vi "占空比.vi"() -> (1 "T1+T2":dbl, 2 "T2":dbl, 3 "T1":dbl)   [LabVIEW 2020]
uses:
  <vilib>/DAQmx/read.llb/DAQmx Read (Counter 1D DBL 1Chan NSamp).vi
  <vilib>/DAQmx/create/channels.llb/DAQmx Create Channel (CI-Pulse Width).vi
  <vilib>/DAQmx/miscellaneous.llb/DAQmx Fill In Error Info.vi
  <vilib>/ptbypt/NI_PtbyPt.lvlib
  <resource>/objmgr/daqmx.rc
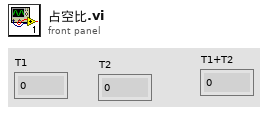
[diagram p1: front panel]
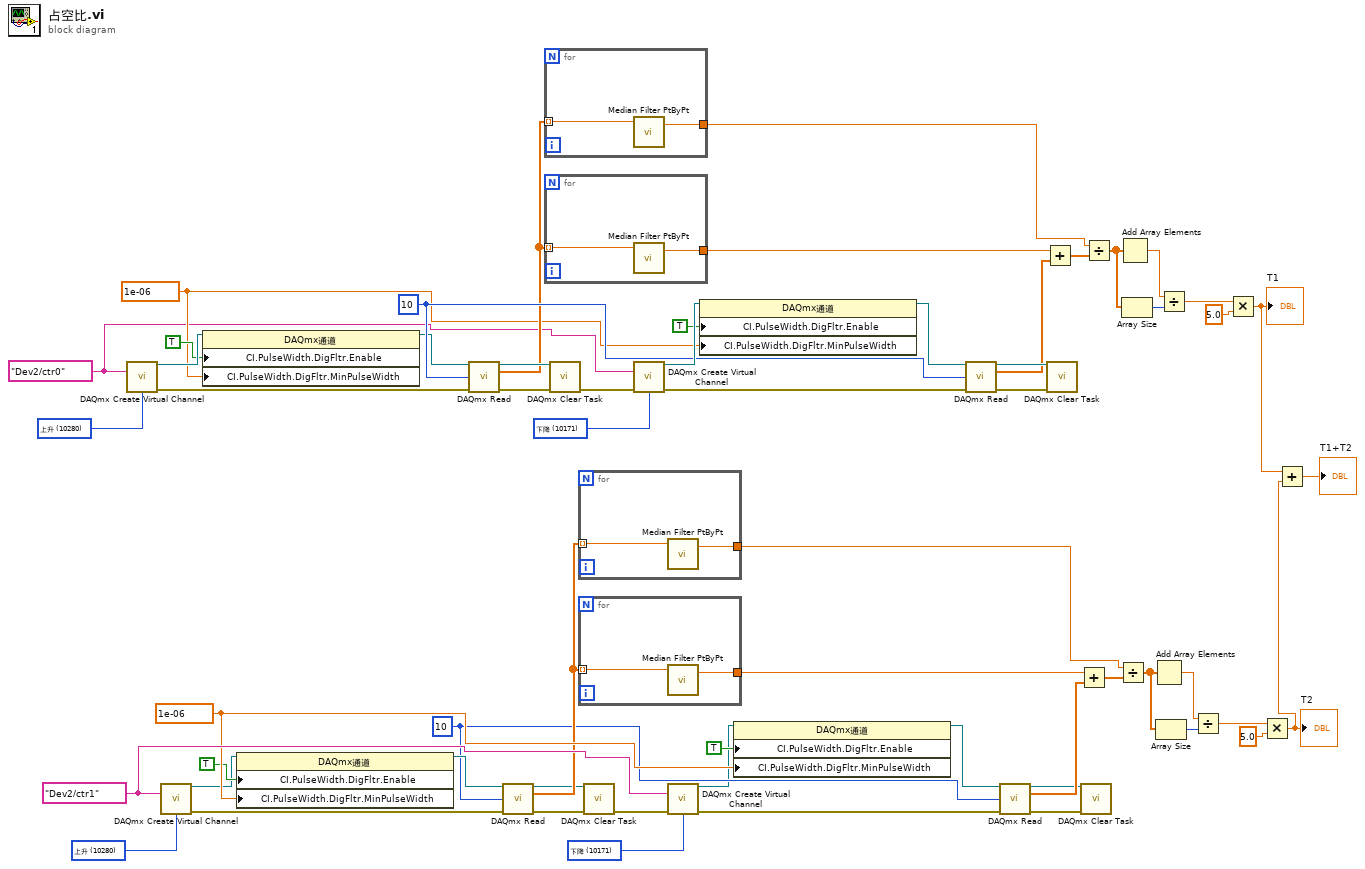
[diagram p0: block diagram]
diagram:
  w30 = 1e-06 ("CI.PulseWidth.DigFltr.MinPulseWidth")
  w15 = 10 ("number of samples per channel")
  w14 = 10280 items=["上升"=10280, "下降"=10171] ("starting edge")
  w13 = 10171 items=["上升"=10280, "下降"=10171] ("starting edge")
  w31 = tag "Dev2/ctr1" ("counter")
  w33 = 1e-06 ("CI.PulseWidth.DigFltr.MinPulseWidth")
  w48 = 10 ("number of samples per channel")
  w49 = 10280 items=["上升"=10280, "下降"=10171] ("starting edge")
  w50 = 10171 items=["上升"=10280, "下降"=10171] ("starting edge")
  w32 = tag "Dev2/ctr0" ("counter")
  n1 = call-poly <vilib>:"DAQmx Create Virtual Channel.vi"("counter"=w32, "starting edge"=w49) -> ("task out"=w59:refnum<k21>, "error out"=w58:errorcluster)  [unwired: 12 in]
  n2 = call-poly <vilib>:"DAQmx Create Virtual Channel.vi"("counter"=w31, "starting edge"=w14) -> ("task out"=w4:refnum<k21>, "error out"=w5:errorcluster)  [unwired: 12 in]
  n3 = property class="DAQmx通道"(reference=w59, "CI.PulseWidth.DigFltr.Enable"=TRUE, "CI.PulseWidth.DigFltr.MinPulseWidth"=w33) -> (reference out=w37:refnum<k21>)  [unwired: 1 in, 1 out]
  n4 = property class="DAQmx通道"(reference=w4, "CI.PulseWidth.DigFltr.Enable"=TRUE, "CI.PulseWidth.DigFltr.MinPulseWidth"=w30) -> (reference out=w26:refnum<k21>)  [unwired: 1 in, 1 out]
  n5 = call-poly <vilib>:"DAQmx Read.vi"("task/channels in"=w37, "number of samples per channel"=w48, "error in"=w58) -> ("task out"=w56:refnum<k21>, "data"=w45:dbl[], "error out"=w57:errorcluster)  [unwired: 10 in]
  n6 = call-poly <vilib>:"DAQmx Read.vi"("task/channels in"=w26, "number of samples per channel"=w15, "error in"=w5) -> ("task out"=w7:refnum<k21>, "data"=w18:dbl[], "error out"=w6:errorcluster)  [unwired: 10 in]
  n7 = for {
    tunnel: w45 -> [w61] mode=indexing
    tunnel: [w60] -> w39
    n8 = call <vilib>:"Median Filter PtByPt.vi"("x"=w61) -> ("Filtered x"=w60:dbl)  [unwired: 3 in, 1 out]
  }
  n9 = for {
    tunnel: w45 -> [w63] mode=indexing
    tunnel: [w62] -> w38
    n10 = call <vilib>:"Median Filter PtByPt.vi"("x"=w63) -> ("Filtered x"=w62:dbl)  [unwired: 3 in, 1 out]
  }
  n11 = call <vilib>:"DAQmx Clear Task.vi"("task in"=w56, "error in"=w57) -> ("error out"=w51:errorcluster)  [unwired: 13 in]
  n12 = for {
    tunnel: w18 -> [w65] mode=indexing
    tunnel: [w64] -> w24
    n13 = call <vilib>:"Median Filter PtByPt.vi"("x"=w65) -> ("Filtered x"=w64:dbl)  [unwired: 3 in, 1 out]
  }
  n14 = for {
    tunnel: w18 -> [w67] mode=indexing
    tunnel: [w66] -> w25
    n15 = call <vilib>:"Median Filter PtByPt.vi"("x"=w67) -> ("Filtered x"=w66:dbl)  [unwired: 3 in, 1 out]
  }
  n16 = call <vilib>:"DAQmx Clear Task.vi"("task in"=w7, "error in"=w6) -> ("error out"=w12:errorcluster)  [unwired: 13 in]
  n17 = call-poly <vilib>:"DAQmx Create Virtual Channel.vi"("counter"=w32, "error in"=w51, "starting edge"=w50) -> ("task out"=w52:refnum<k21>, "error out"=w53:errorcluster)  [unwired: 11 in]
  n18 = call-poly <vilib>:"DAQmx Create Virtual Channel.vi"("counter"=w31, "error in"=w12, "starting edge"=w13) -> ("task out"=w11:refnum<k21>, "error out"=w10:errorcluster)  [unwired: 11 in]
  n19 = property class="DAQmx通道"(reference=w52, "CI.PulseWidth.DigFltr.Enable"=TRUE, "CI.PulseWidth.DigFltr.MinPulseWidth"=w33) -> (reference out=w35:refnum<k21>)  [unwired: 1 in, 1 out]
  n20 = property class="DAQmx通道"(reference=w11, "CI.PulseWidth.DigFltr.Enable"=TRUE, "CI.PulseWidth.DigFltr.MinPulseWidth"=w30) -> (reference out=w28:refnum<k21>)  [unwired: 1 in, 1 out]
  n21 = call-poly <vilib>:"DAQmx Read.vi"("task/channels in"=w35, "number of samples per channel"=w48, "error in"=w53) -> ("task out"=w55:refnum<k21>, "data"=w47:dbl[], "error out"=w54:errorcluster)  [unwired: 10 in]
  n22 = call-poly <vilib>:"DAQmx Read.vi"("task/channels in"=w28, "number of samples per channel"=w15, "error in"=w10) -> ("task out"=w8:refnum<k21>, "data"=w16:dbl[], "error out"=w9:errorcluster)  [unwired: 10 in]
  n23 = Add(x=w38, y=w47) -> (x+y=w46:dbl[])
  n24 = call <vilib>:"DAQmx Clear Task.vi"("task in"=w55, "error in"=w54) -> ()  [unwired: 13 in, 1 out]
  n25 = Add(x=w25, y=w16) -> (x+y=w17:dbl[])
  n26 = call <vilib>:"DAQmx Clear Task.vi"("task in"=w8, "error in"=w9) -> ()  [unwired: 13 in, 1 out]
  n27 = Divide(x=w39, y=w46) -> (x/y=w44:dbl[])
  n28 = Divide(x=w24, y=w17) -> (x/y=w19:dbl[])
  n29 = Add Array Elements(numeric array=w44) -> (sum=w43:dbl)
  n30 = Array Size(array=w44) -> (size(s)=w42:i32)
  n31 = Add Array Elements(numeric array=w19) -> (sum=w20:dbl)
  n32 = Array Size(array=w19) -> (size(s)=w21:i32)
  n33 = Divide(x=w43, y=w42) -> (x/y=w41:dbl)
  n34 = Divide(x=w20, y=w21) -> (x/y=w22:dbl)
  n35 = Multiply(x=w41, y=5.0) -> (x*y=w3:dbl)
  "T1" <- w3
  n36 = Multiply(x=w22, y=5.0) -> (x*y=w2:dbl)
  "T2" <- w2
  n37 = Add(x=w3, y=w2) -> (x+y=→"T1+T2":dbl)
